vi "[FGV] Template.vi"(8 "error in (no error)":errorcluster, 9 "Image Name Array":string[](array[string]), 10 "Image Array":T1[](array[typedef]), 11 "Command":enum16{"Initialize", "Save", "Read"}(ring)) -> (0 "error out":errorcluster, 2 "Image Name Array":string[](array[string]), 3 "Image Array":T1[](array[typedef]))   [LabVIEW 2019]
uses:
  <vilib>/vision/Image Controls.llb/IMAQ Image.ctl
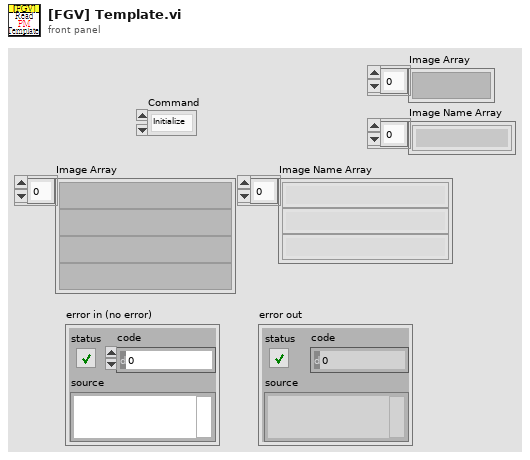
[diagram p1: front panel]
types:
  T1 = typedef "IMAQ Image.ctl" = refnum<image>
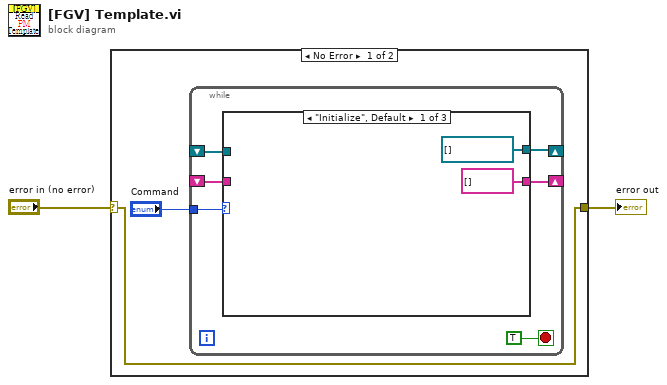
[diagram p0: block diagram]
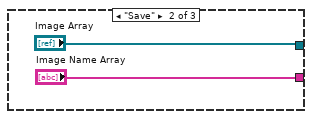
[diagram p2: hidden frame]
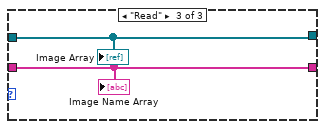
[diagram p3: hidden frame]
diagram:
  n1 = case shown="No Error" "error in (no error)" {
    selector: "error in (no error)" -> [w3 w17]
    tunnel: [w3 w17] -> w1
    frame No Error {
      n2 = while {
        tunnel: "Command" -> [w10]
        shift-right: [w8] -> _
        shift-left: _ -> [w7]
        shift-right: [w6] -> _
        shift-left: _ -> [w5]
        stop <- TRUE stop-if-true
        n3 = case shown="\"Initialize\", Default" w10 {
          tunnel: [T1[] [] ("Image Array") "Image Array" w16] -> w8
          tunnel: w7 -> [_ _ w16]
          tunnel: [string[] [] ("Image Name Array") "Image Name Array" w15] -> w6
          tunnel: w5 -> [_ _ w15]
          frame "Initialize", Default {
          }
          frame "Save" {
          }
          frame "Read" {
            "Image Array" <- w16
            "Image Name Array" <- w15
          }
        }
      }
    }
    frame Error {
    }
  }
  "error out" <- w1
